vi "myRIO v1.0 Close.vi"(8 "error in (no error)":errorcluster, 11 "myRIO FPGA Ref In":T1) -> (0 "error out":errorcluster)   [LabVIEW 2021]
uses:
  <vilib>/myRIO/Common/Instrument Driver Framework/Utilities/typedefs/Generic FPGA Reference.ctl
  <vilib>/myRIO/Common/Instrument Driver Framework/Utilities/typedefs/Ref Counter Action Enum.ctl
  <vilib>/myRIO/Common/Instrument Driver Framework/Utilities/typedefs/FPGA Ref Manager Action Enum.ctl
  <vilib>/FPGAPlugInAG/Dynamic/niLvFpga_Close_Dynamic.vi
  <vilib>/rvi/interface/nirviCloseFPGA/nirviCloseFPGA.xnode
panel:
  # "This VI closes the reference to the FPGA target on the \nmyRIO v1.0 hardware. Please see the Block Diagram for details."
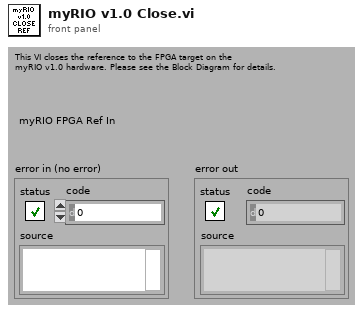
[diagram p1: front panel]
types:
  T1 = typedef "Generic FPGA Reference.ctl" = refnum<k20>
  T2 = typedef "FPGA Ref Manager Action Enum.ctl" = enum16{"Get", "Set", "Reset"}
  T3 = typedef "Ref Counter Action Enum.ctl" = enum16{"Set", "Get", "Increment", "Decrement"}
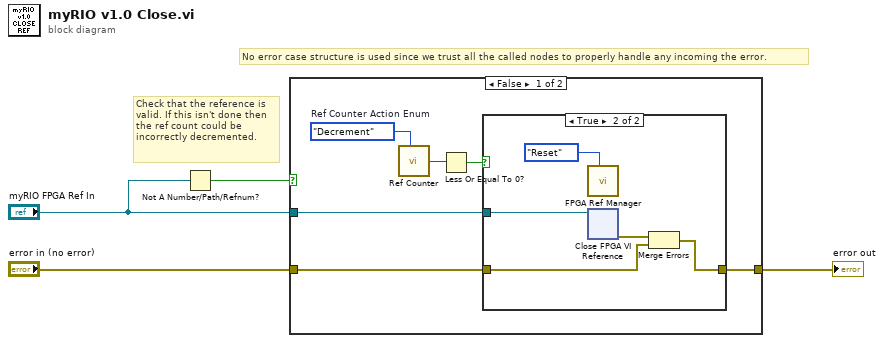
[diagram p0: block diagram]
diagram:
  # "No error case structure is used since we trust all the called nodes to properly handle any incoming the error."
  # "Check that the reference is valid. If this isn't done then the ref count could be incorrectly decremented."
  n1 = Not A Number/Path/Refnum?(number/path/refnum="myRIO FPGA Ref In") -> (NaN/Path/Refnum?=w4:bool)
  n2 = case shown="False" w4 {
    tunnel: "myRIO FPGA Ref In" -> [w7 _]
    tunnel: "error in (no error)" -> [w6 w17]
    tunnel: [w5 w17] -> w1
    frame False {
      w10 = Ref_Counter_Action_Enum."Decrement"  # Ref Counter Action Enum
      n3 = call <vilib>:"Ref Counter.vi"("Ref Counter Action Enum"=w10) -> ("Ref Count out"=w9:u32)  [unwired: 1 in]
      n4 = Less Or Equal To 0?(x=w9) -> (x <= 0?=w8:bool)
      n5 = case shown="True" w8 {
        tunnel: w6 -> [w11 w12]
        tunnel: [w11 w13] -> w5
        tunnel: w7 -> [_ w15]
        frame False {
        }
        frame True {
          n6 = call <vilib>:"FPGA Ref Manager.vi"("Action"=FPGA_Ref_Manager_Action_Enum."Reset") -> ()  [unwired: 8 in, 2 out]
          n7 = xnode "Close FPGA VI Reference"("FPGA VI Reference In"=w15) -> ("error out"=w16:errorcluster)  [unwired: 1 in]
          n8 = Merge Errors(w16, w12) -> (w13:errorcluster)
        }
      }
    }
    frame True {
    }
  }
  "error out" <- w1
